vi "释放通道后申请通道_CLK.vi"(8 "error in":errorcluster) -> (0 "error out":errorcluster)   [LabVIEW 2015]
uses:
  Global/SeverGlobal.vi
panel:
  out "ack":string
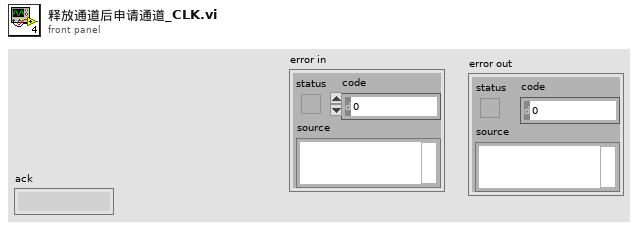
[diagram p1: front panel]
types:
  T1 = enum16{"open", "replace", "create", "open or create", "replace or create", "replace or create with confirmation"}
  T2 = typedef "响应消息头.ctl" = string
  T3 = cluster{"TCP Ref":refnum<k5>, "IP":string, "userName":string, "IN":u16, "OUT":u16, "time":u32}[]
  T4 = typedef "队列.ctl" = cluster{"COM1":refnum<queue>, "COM2":refnum<queue>, "COM3":refnum<queue>, "COM4":refnum<queue>, "OUT1":refnum<queue>, "OUT2":refnum<queue>, "OUT3":refnum<queue>, "OUT4":refnum<queue>, "OUT5":refnum<queue>, "OUT6":refnum<queue>, "OUT7":refnum<queue>, "OUT8":refnum<queue>}
  T5 = cluster{"TCP Ref":refnum<k5>, "Broadcast":refnum<k5>, "TF Ref":refnum<k5>, "IP":string, "port":u16, "userName":string, "passWord":string, "authority":string}[]
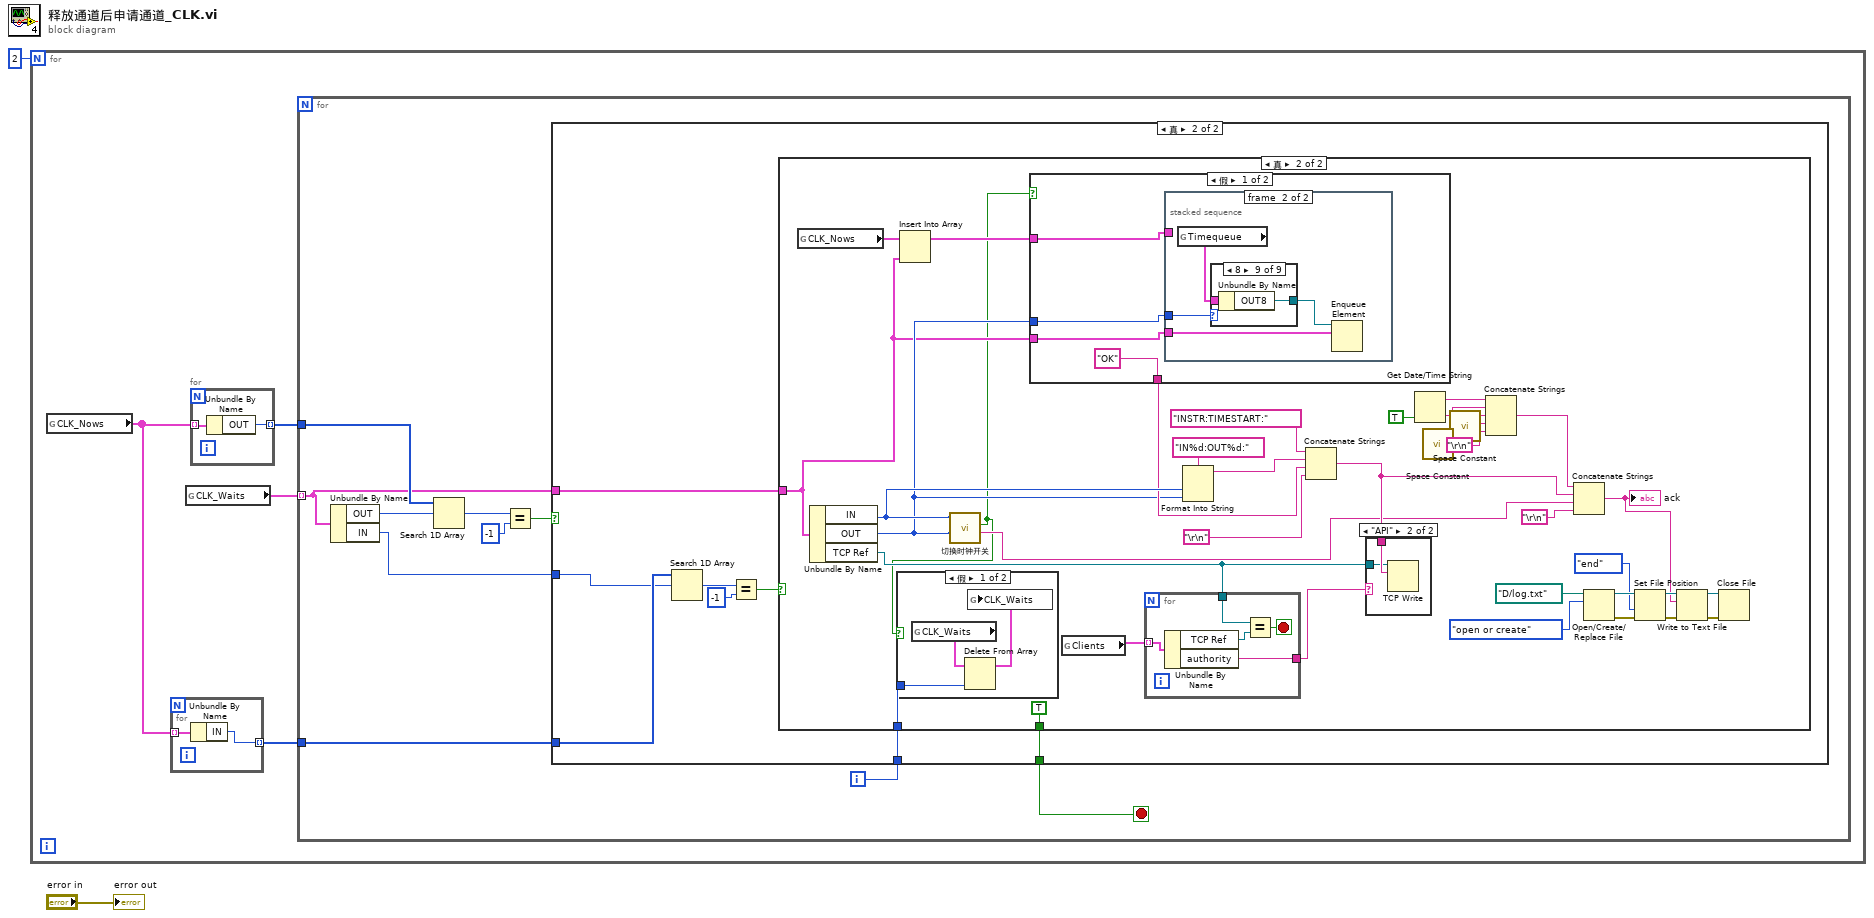
[diagram p0: block diagram]
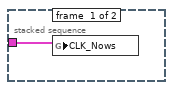
[diagram p5: hidden frame]
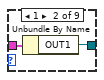
[diagram p7: hidden frame]
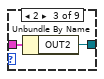
[diagram p8: hidden frame]
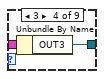
[diagram p9: hidden frame]
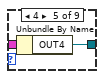
[diagram p10: hidden frame]
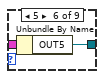
[diagram p11: hidden frame]
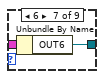
[diagram p12: hidden frame]
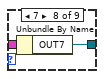
[diagram p13: hidden frame]
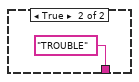
[diagram p14: hidden frame]
diagram:
  n1 = for {
    N: 2 -> [_]
    n2 = global read "SeverGlobal.vi" "CLK_Nows"() -> (w4:T3)
    n3 = for {
      tunnel: w4 -> [w8] mode=indexing
      tunnel: [w7] -> w3 mode=indexing
      n4 = Unbundle By Name(w8) -> ("IN"=w7:u16)
    }
    n5 = global read "SeverGlobal.vi" "CLK_Waits"() -> (w6:T3)
    n6 = for {
      tunnel: w4 -> [w100] mode=indexing
      tunnel: [w99] -> w5 mode=indexing
      n7 = Unbundle By Name(w100) -> ("OUT"=w99:u16)
    }
    n8 = for {
      tunnel: w6 -> [w11] mode=indexing
      tunnel: w5 -> [w15]
      tunnel: w3 -> [w13]
      i -> [w9]
      stop <- w10 stop-if-true
      n9 = Unbundle By Name(w11) -> ("OUT"=w16:u16, "IN"=w12:u16)
      n10 = Search 1D Array(1D array=w15, element=w16) -> (index of element=w18:i32)  [unwired: 1 in]
      n11 = Equal?(x=w18, y=-1) -> (x = y?=w14:bool)
      n12 = case shown="真" w14 {
        tunnel: w13 -> [_ w24]
        tunnel: w12 -> [_ w19]
        tunnel: w11 -> [_ w22]
        tunnel: [_ w21] -> w10
        tunnel: w9 -> [_ w20]
        frame False {
          # "OUT冲突，不作为"
        }
        frame True {
          n13 = Search 1D Array(1D array=w24, element=w19) -> (index of element=w25:i32)  [unwired: 1 in]
          n14 = Equal?(x=w25, y=-1) -> (x = y?=w23:bool)
          n15 = case shown="真" w23 {
            tunnel: w22 -> [_ w28]
            tunnel: [_ TRUE] -> w21
            tunnel: w20 -> [_ w60]
            frame False {
              # "IN冲突，不作为"
            }
            frame True {
              n16 = global read "SeverGlobal.vi" "CLK_Nows"() -> (w62:T3)
              n17 = Unbundle By Name(w28) -> ("IN"=w55:u16, "OUT"=w29:u16, "TCP Ref"=w53:refnum<k5>)
              n18 = Insert Into Array(array=w62, new element=w28) -> (w30:T3)  [unwired: 1 in]
              n19 = call "切换时钟开关.vi"("OUT"=w29, "IN"=w55) -> ("ask"=w32:string, "Isfailed"=w27:bool)  [unwired: 7 in, 1 out]
              n20 = case shown="假" w27 {
                tunnel: w60 -> [w64 _]
                frame False {
                  n21 = global read "SeverGlobal.vi" "CLK_Waits"() -> (w65:T3)
                  n22 = Delete From Array(array=w65, index=w64) -> (array with subset deleted=w63:T3)  [unwired: 1 in, 1 out]
                  n23 = global write "SeverGlobal.vi" "CLK_Waits"(w63) -> ()
                }
                frame True {
                }
              }
              n24 = case shown="假" w27 {
                tunnel: ["OK" ("format string") "TROUBLE" ("format string")] -> w51
                tunnel: w30 -> [w68 _]
                tunnel: w29 -> [w67 _]
                tunnel: w28 -> [w66 _]
                frame False {
                  n25 = stacked-sequence {
                    tunnel: w68 -> [w70 _]
                    tunnel: w67 -> [_ w72]
                    tunnel: w66 -> [_ w71]
                    frame #0 {
                      n26 = global write "SeverGlobal.vi" "CLK_Nows"(w70) -> ()
                    }
                    frame #1 {
                      n27 = global read "SeverGlobal.vi" "Timequeue"() -> (w74:T4)
                      n28 = case shown="8" w72 {
                        tunnel: w74 -> [_ w76 w78 w80 w82 w84 w86 w88 w90]
                        tunnel: [_ w75 w77 w79 w81 w83 w85 w87 w89] -> w73
                        frame 0, Default {
                        }
                        frame 1 {
                          n29 = Unbundle By Name(w76) -> ("OUT1"=w75:refnum<queue>)
                        }
                        frame 2 {
                          n30 = Unbundle By Name(w78) -> ("OUT2"=w77:refnum<queue>)
                        }
                        frame 3 {
                          n31 = Unbundle By Name(w80) -> ("OUT3"=w79:refnum<queue>)
                        }
                        frame 4 {
                          n32 = Unbundle By Name(w82) -> ("OUT4"=w81:refnum<queue>)
                        }
                        frame 5 {
                          n33 = Unbundle By Name(w84) -> ("OUT5"=w83:refnum<queue>)
                        }
                        frame 6 {
                          n34 = Unbundle By Name(w86) -> ("OUT6"=w85:refnum<queue>)
                        }
                        frame 7 {
                          n35 = Unbundle By Name(w88) -> ("OUT7"=w87:refnum<queue>)
                        }
                        frame 8 {
                          n36 = Unbundle By Name(w90) -> ("OUT8"=w89:refnum<queue>)
                        }
                      }
                      n37 = Enqueue Element(queue=w73, element=w71) -> ()  [unwired: 2 in, 3 out]
                    }
                  }
                }
                frame True {
                }
              }
              n38 = global read "SeverGlobal.vi" "Clients"() -> (w54:T5)
              n39 = for {
                tunnel: w54 -> [w98] mode=indexing
                tunnel: w53 -> [w96]
                tunnel: [w94] -> w52
                stop <- w95 stop-if-true
                n40 = Unbundle By Name(w98) -> ("TCP Ref"=w97:refnum<k5>, "authority"=w94:string)
                n41 = Equal?(x=w96, y=w97) -> (x = y?=w95:bool)
              }
              n42 = Format Into String(format string="IN%d:OUT%d:", w55, w29) -> (resulting string=w57:string)  [unwired: 2 in, 1 out]
              n43 = Concatenate Strings(T2 "INSTR:TIMESTART:" ("Combo Box"), w57, w51, "\r\n") -> (w43:string)
              n44 = case shown="\"API\"" w52 {
                tunnel: w43 -> [_ w93]
                tunnel: w53 -> [_ w92]
                frame "False", Default {
                }
                frame "API" {
                  n45 = TCP Write(connection ID=w92, data in=w93) -> ()  [unwired: 2 in, 3 out]
                }
              }
              n46 = Get Date/Time String(want seconds? (F)=TRUE ("需要秒？(F)")) -> (date string=w45:string, time string=w46:string)  [unwired: 2 in]
              n47 = call <vilib>:"Space Constant.vi"() -> ("String"=w47:string)
              n48 = call <vilib>:"Space Constant.vi"() -> ("String"=w48:string)
              n49 = Concatenate Strings(w45, w47, w46, w48, "\r\n") -> (w50:string)
              n50 = Concatenate Strings(w50, w43, w32, "\r\n") -> (w33:string)
              "ack" <- w33
              n51 = Open/Create/Replace File(file path (use dialog)=path "D:/log.txt" ("文件（使用对话框）"), operation (0:open)=T1."open or create" ("操作(0:open)")) -> (refnum out=w39:refnum<file>, error out=w40:errorcluster)  [unwired: 4 in, 1 out]
              n52 = Set File Position(refnum=w39, from (0:start)=enum16{"start", "end", "current"}."end" ("自（0:起始）"), error in=w40) -> (refnum out=w41:refnum<file>, error out=w42:errorcluster)  [unwired: 1 in]
              n53 = Write to Text File(file (use dialog)=w41, text=w33, error in=w42) -> (refnum out=w37:refnum<file>, error out=w36:errorcluster)  [unwired: 1 in, 1 out]
              n54 = Close File(refnum=w37, error in=w36) -> ()  [unwired: 2 out]
            }
          }
        }
      }
    }
  }
  "error out" <- "error in"
